vi "GetReplyTo.vi"(8 "error in (no error)":errorcluster, 11 "service in":refnum<class "IcmMessageService.lvclass">) -> (0 "error out":errorcluster, 2 "reply to":string, 3 "service out":refnum<class "IcmMessageService.lvclass">)   [LabVIEW 2017, in "IcmMessageService.lvclass"]
doc: "Returns the full name of the service as recognized by the message bus. Use this name for the purpose of routing messages."
uses:
  <vilib>/addons/InsightCM/MessageBus/MessageService/IcmMessageService.lvclass
  <vilib>/addons/InsightCM/MessageBus/MessageService/IcmMessageService.lvclass/IcmMessageService.ctl
  C:/Program Files (x86)/National Instruments/LabVIEW 2017/vi.lib/addons/InsightCM/Binaries/LabviewMessageAdapter.dll
  Binaries/LabviewMessageAdapter.dll
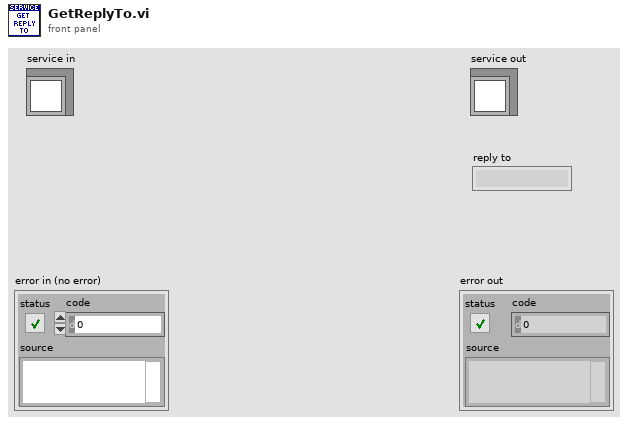
[diagram p1: front panel]
types:
  T1 = typedef "MessageServiceDvr.ctl" = refnum<data-value>
  T2 = typedef "MessageServiceData.ctl" = cluster{"Service":refnum<k24>}
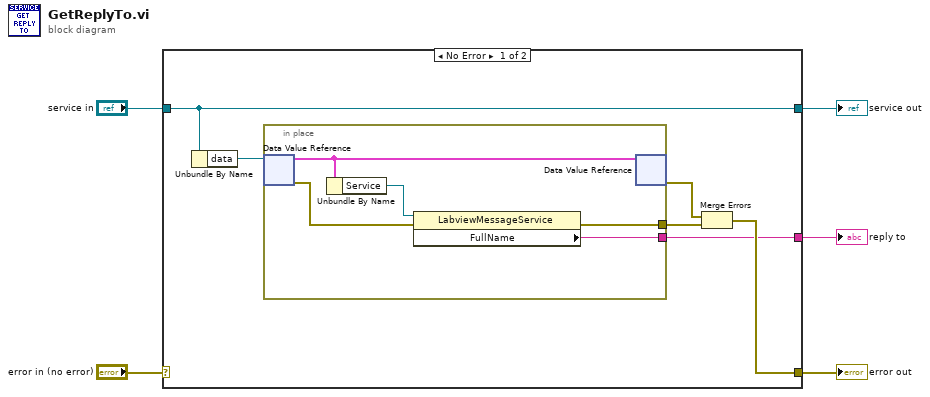
[diagram p0: block diagram]
diagram:
  n1 = case shown="No Error" "error in (no error)" {
    selector: "error in (no error)" -> [_ w18]
    tunnel: [w7 w18] -> w5
    tunnel: [w11 w17] -> w3
    tunnel: "service in" -> [w11 w17]
    tunnel: [w6 _] -> w1
    frame No Error {
      n2 = Unbundle By Name(w11) -> ("data"=w10:T1)
      n3 = in-place {
        in-place-border: [w13] -> w8
        in-place-border: [w12] -> w6
        n4 = in-place-dvr #1(w10) -> (w16:T2, w15:errorcluster)
        n5 = Unbundle By Name(w16) -> ("Service"=w14:refnum<k24>)
        n6 = property class="LabviewMessageService"(reference=w14, error in=w15) -> (error out=w13:errorcluster, "FullName"=w12:string)  [unwired: 1 out]
        n7 = in-place-dvr #1(w16) -> (w9:errorcluster)  [unwired: 1 out]
      }
      n8 = Merge Errors(w9, w8) -> (w7:errorcluster)
    }
    frame Error {
    }
  }
  "error out" <- w5
  "service out" <- w3
  "reply to" <- w1
